vi "manual middle-man to plc barcode print.vi"(8 "error in":errorcluster, 10 "station default states":T1[](array[typedef]) {"LIN INFO"."NAD" format="%.0x"; "LIN INFO"."ADCS LIN"."HW select" items=["NI-XNET", "NI-CAN"]; "LVDT Status"."LVDT's stored config"."Lower Limit" format="%.2f"; "LVDT Status"."LVDT's stored config"."Upper Limit" format="%.2f"; "Store Data"."Sun Shade Open Force Limits"."Variance" format="%.2g"; "Store Data"."Sun Shade Open Force Limits"."Truncation End" format="%.2g"; "Store Data"."Sun Shade Open Force Limits"."Truncation Start" format="%.2g"; "Store Data"."Sun Shade Open Force Limits"."Avg Max" format="%.2g"; "Store Data"."Sun Shade Open Force Limits"."Avg Min" format="%.2g"; "Store Data"."Sun Shade Open Force Limits"."Overall Max" format="%.2g"; "Store Data"."Sun Shade Open Force Limits"."Overall Min" format="%.2g"; "Store Data"."Sun Shade Close Force Limits"."Variance" format="%.2g"; "Store Data"."Sun Shade Close Force Limits"."Truncation End" format="%.2g"; "Store Data"."Sun Shade Close Force Limits"."Truncation Start" format="%.2g"; "Store Data"."Sun Shade Close Force Limits"."Avg Max" format="%.2g"; "Store Data"."Sun Shade Close Force Limits"."Avg Min" format="%.2g"; "Store Data"."Sun Shade Close Force Limits"."Overall Max" format="%.2g"; "Store Data"."Sun Shade Close Force Limits"."Overall Min" format="%.2g"}, 11 "exit program ref":refnum<vi>) -> (0 "error out":errorcluster)   [LabVIEW 2018]
uses:
  05.UserVI's/BarCode/typedefs/barcode printer types.ctl
  05.UserVI's/BarCode/typedefs/barcode format params.ctl
  02.Type Def's/EOL Module Info Control.ctl
  <vilib>/Platform/dataskt.llb/DataSocket Reference Type.ctl
  05.UserVI's/type defs/plc path and tag.ctl
  02.Type Def's/station plc read string tags.ctl
  02.Type Def's/station plc read boolean tags.ctl
  05.UserVI's/type defs/EOL Motor Type.ctl
  05.UserVI's/type defs/RAP Signal Control.ctl
  05.UserVI's/type defs/Communication with Motors.ctl
  02.Type Def's/All Communication Types.ctl
  05.UserVI's/type defs/EOL Part Setup.ctl
  02.Type Def's/All Motions.ctl
  02.Type Def's/EOL Switch Max Min Check Cluster.ctl
  02.Type Def's/EOL Switch Value Configuration Cluster.ctl
  02.Type Def's/All Switch Configuration Cluster.ctl
  05.UserVI's/type defs/17x Sunshade Limts Seq.ctl
  02.Type Def's/Pass Fail Control.ctl
  05.UserVI's/type defs/17x AP Data Type.ctl
  05.UserVI's/type defs/17x Audit Motion Data Seq Control.ctl
  02.Type Def's/EOL Motion Database Table.ctl
  05.UserVI's/sequence/type defs/Sequence Info.ctl
  02.Type Def's/station nvh config.ctl
  02.Type Def's/station rs232 port map.ctl
  02.Type Def's/station ethernet address map.ctl
  02.Type Def's/station paths.ctl
  02.Type Def's/EOL Save Module Test Data Control.ctl
  05.UserVI's/type defs/EOL Global Digital Input Control.ctl
  02.Type Def's/station DI map.ctl
  02.Type Def's/Screen Motion Data.ctl
  02.Type Def's/station motion data indicator.ctl
  02.Type Def's/lvdt name val pair.ctl
  02.Type Def's/station hmi.ctl
  02.Type Def's/individual station status.ctl
  02.Type Def's/control refs.ctl
  05.UserVI's/type defs/EOL LVDT's Check Controller.ctl
  05.UserVI's/Lambda Power/power supply types.ctl
  05.UserVI's/LVDT's/lvdt precision.ctl
  02.Type Def's/main state cluster.ctl
  02.Type Def's/sequence state.ctl
  03.Inalfa LIN/LIN Device.ctl
  <vilib>/CMC.AME/Inalfa ADCS/Ctl'Def/ADCS_LIN info.ctl
  C:/Program Files (x86)/National Instruments/LabVIEW 2018/vi.lib/CMC.AME/_Inalfa TS LIN_internal_deps/Interop.TSMasterAPI.dll
  Program Files (x86)/National Instruments/LabVIEW 2018/vi.lib/CMC.AME/_Inalfa TS LIN_internal_deps/Interop.TSMasterAPI.dll
  02.Type Def's/station LIN config.ctl
  02.Type Def's/misc station config.ctl
  Sub'VIs/Type Def's/Config Info.ctl
panel:
  # "Sunroof Barcode"
  # "Pallet Number"
  # "Part Type"
  # "Application Status"
  # "Current Step"
  # "Cycle Time"
  # "Pass / Fail"
  # "Shade Close"
  # "Actual Data"
  # "Limits"
  # "Avg Current"
  # "Run Time"
  # "Speed"
  # "Noise Test"
  # "Position"
  # "Shade Open"
  # "Actual Data"
  # "Limits"
  # "Avg Current"
  # "Run Time"
  # "Speed"
  # "Noise Test"
  # "Position"
  # "Vent Close"
  # "Actual Data"
  # "Limits"
  # "Avg Current"
  # "Run Time"
  # "Speed"
  # "Noise Test"
  # "Position"
  # "Vent Open"
  # "Actual Data"
  # "Limits"
  # "Avg Current"
  # "Run Time"
  # "Speed"
  # "Noise Test"
  # "Position"
  # "Slide Close"
  # "Actual Data"
  # "Limits"
  # "Avg Current"
  # "Run Time"
  # "Speed"
  # "Noise Test"
  # "Position"
  # "Slide Open"
  # "Actual Data"
  # "Limits"
  # "Avg Current"
  # "Run Time"
  # "Speed"
  # "Noise Test"
  # "Position"
  # "Min"
  # "N"
  # "Min"
  # "Start"
  # "N"
  # "Max"
  # "N"
  # "Max"
  # "N"
  # "End"
  # "Min"
  # "N"
  # "Min"
  # "Start"
  # "N"
  # "Max"
  # "N"
  # "Max"
  # "N"
  # "End"
  # "Min"
  # "Max"
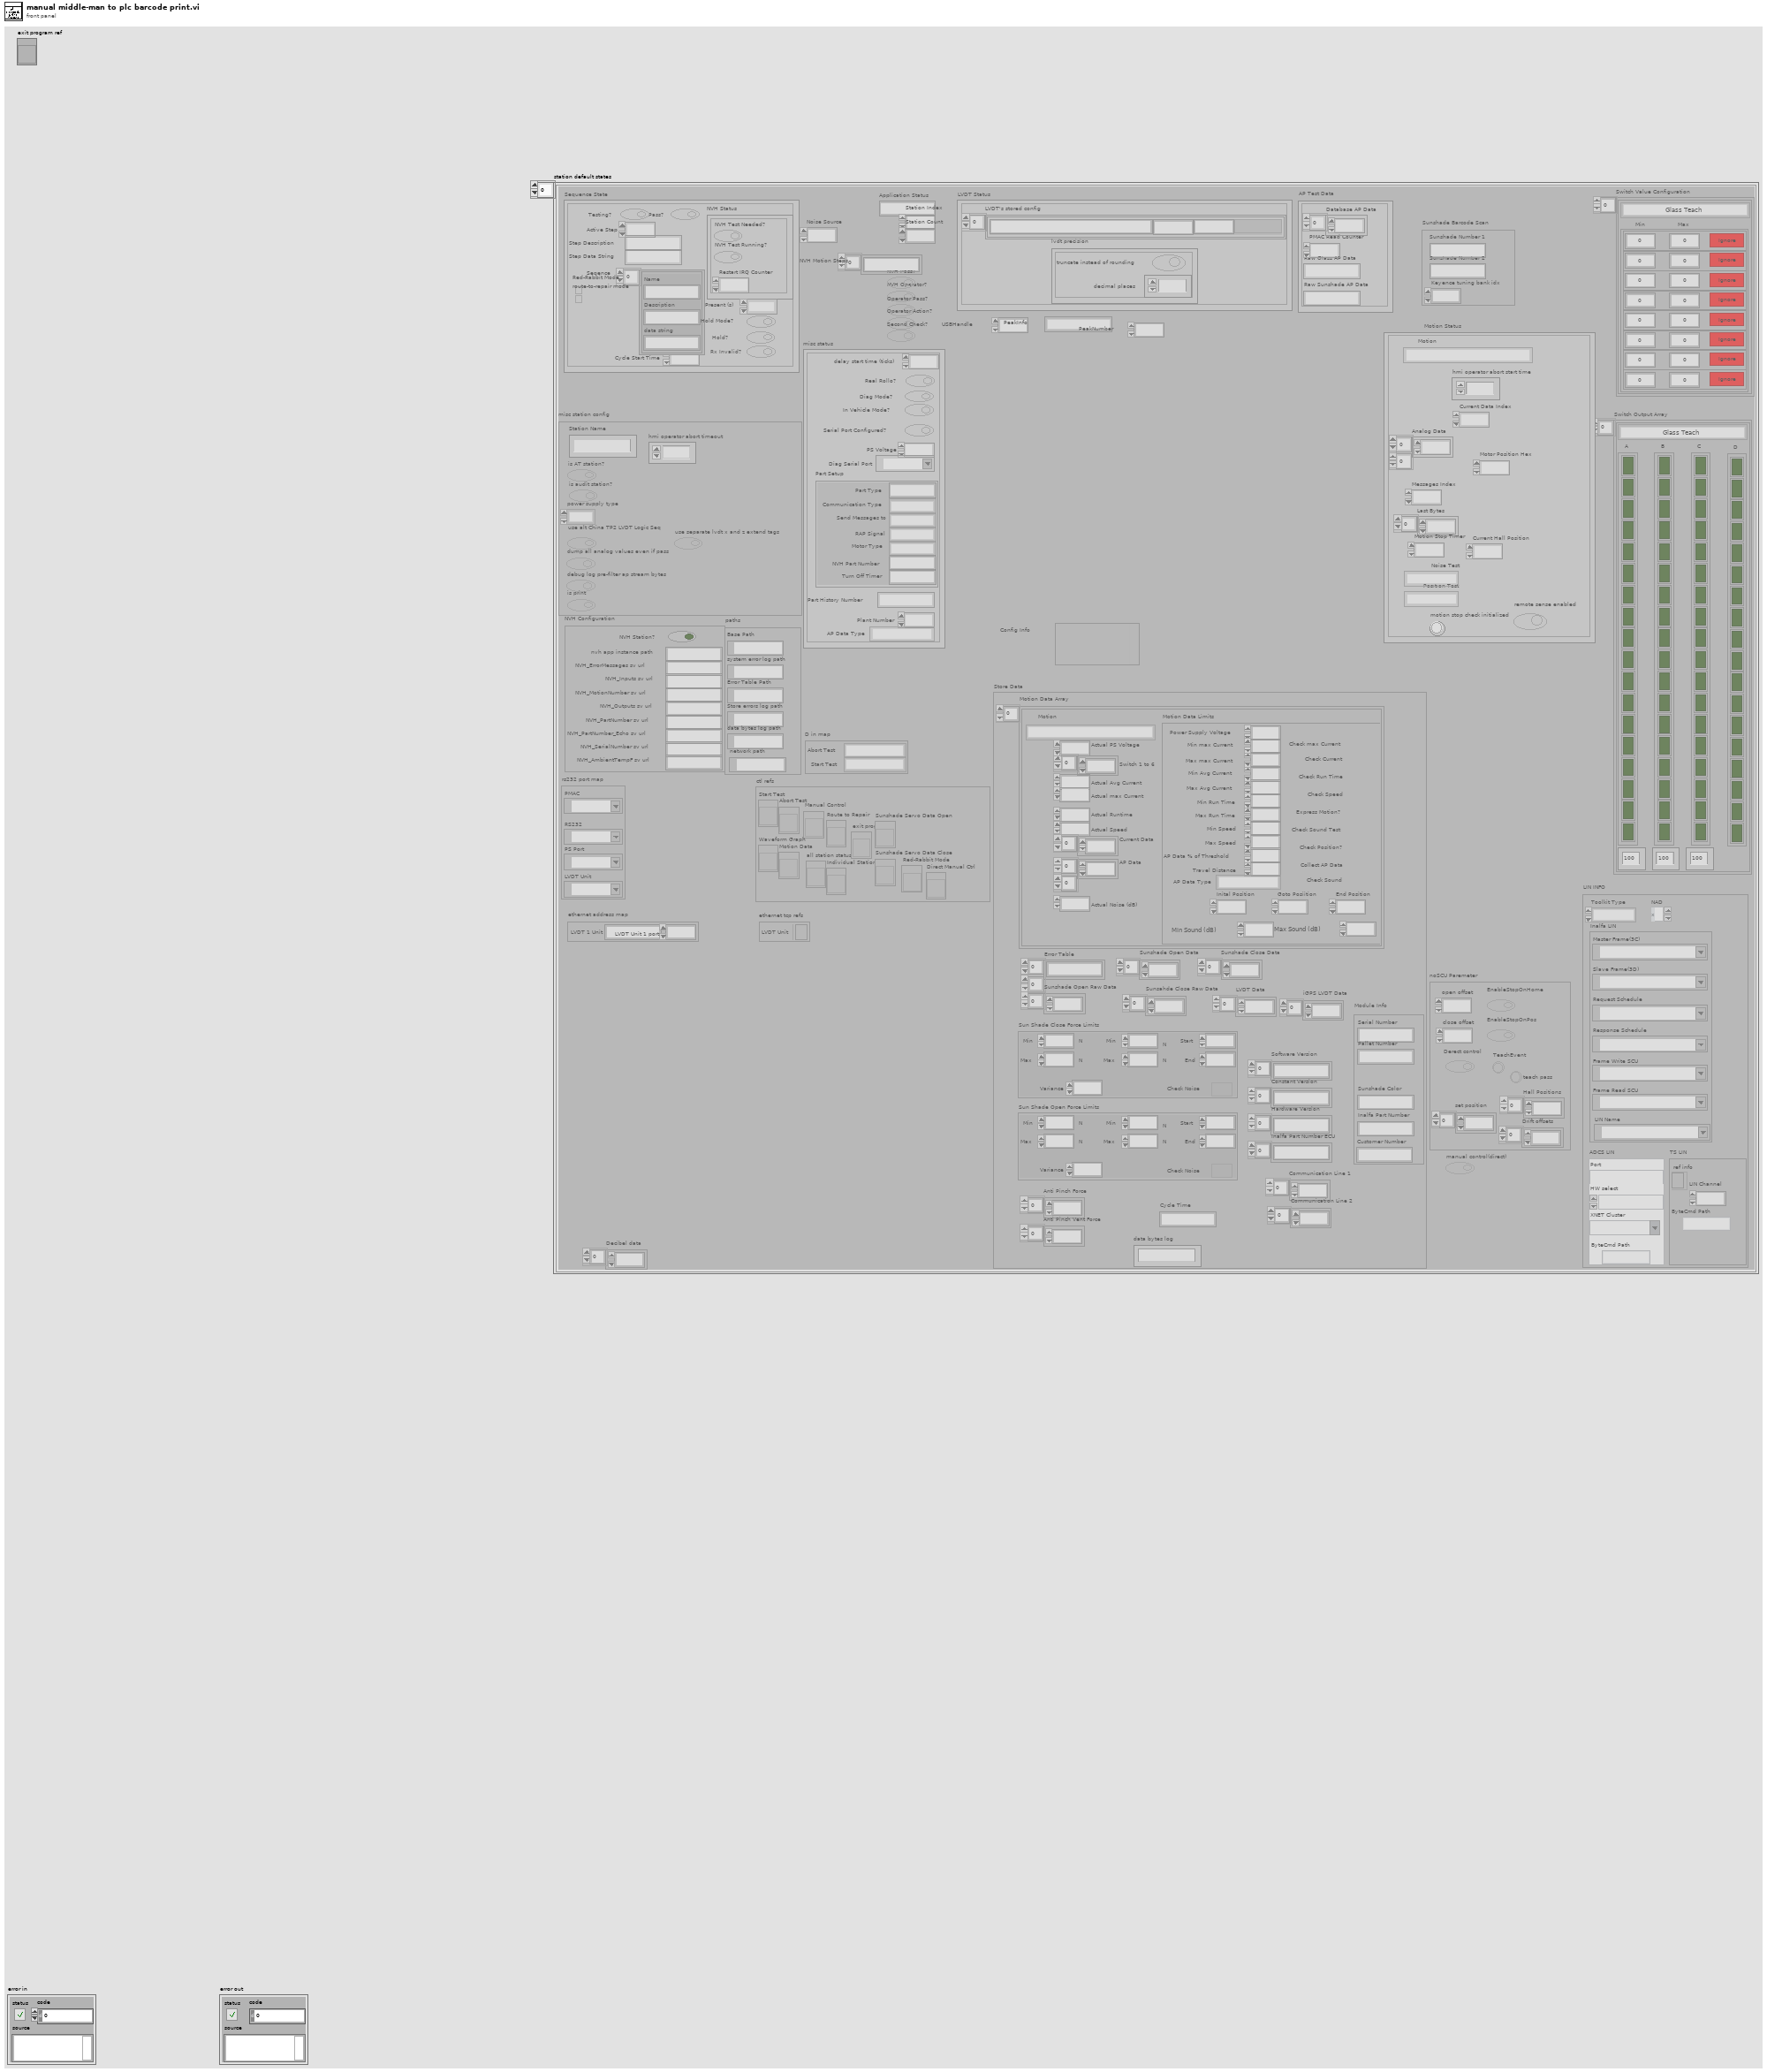
[diagram p1: front panel]
types:
  T1 = typedef "main state cluster.ctl" = cluster{"Application Status":string, "Switch Output Array":T2[], "Switch Value Configuration":T4[], "NVH Configuration":T6, "rs232 port map":T7, "ethernet address map":T8, "paths":T9, "Station Index":i32, "Station Count":i32, "Store Data":T10, "D in map":T16, "ctl refs":T18, "misc station config":T19, "ethernet tcp refs":cluster{"LVDT Unit":refnum<k5>}, "Sunshade Barcode Scan":cluster{"Sunshade Number 2":string, "Sunshade Number 1":string, "Keyence tuning bank idx":i32}, "AP Test Data":cluster{"Raw Sunshade AP Data":string, "Raw Glass AP Data":string, "PMAC Read Counter":dbl, "Database AP Data":dbl[]}, "Motion Status":cluster{"hmi operator abort start time":u32, "Current Data Index":i32, "Analog Data":sgl[][], "Motor Position Hex":u16, "Messages Index":u16, "Last Bytes":u8[], "Current Hall Position":i16, "Motion Stop Timer":u32, "Position Test":T21, "Noise Test":T21, "motion stop check initialized":bool, "remote sense enabled":bool, "Motion":T3}, "LVDT Status":cluster{"LVDT's stored config":T22[], "lvdt precision":T23}, "Sequence State":T24, "misc status":cluster{"delay start time (ticks)":u32, "In Vehicle Mode?":bool, "Diag Mode?":bool, "Serial Port Configured?":bool, "PS Voltage":dbl, "Diag Serial Port":refnum<visa-resource-name>, "Part Setup":T26, "Part History Number":string, "Plant Number":u8, "AP Data Type":T13, "Real Rollo?":bool}, "NVH Operator?":bool, "NVH Pass?":bool, "Operator Pass?":bool, "Operator Action?":bool, "Noise Source":u32, "USBHandle":i32, "PeakInfo":string, "PeakNumber":i32, "NVH Motion Steps":string[], "Second Check?":bool, "Decibel data":dbl[], "noSCU Paremeter":cluster{"EnableStopOnHome":bool, "EnableStopOnPos":bool, "TeachEvent":bool, "open offset":i32, "close offset":i32, "Derect control":bool, "set position":i32[], "teach pass ":bool, "Drift offsets":i32[], "Hall Positions":i32[]}, "manual control(direct)":bool, "LIN INFO":T31, "Config Info":T34}
  T2 = typedef "All Switch Configuration Cluster.ctl" = cluster{"All Motions":T3, "A":bool[], "B":bool[], "C":bool[], "D":bool[], "A activation time (ms)":u32, "B activation time (ms)":u32, "C activation time (ms)":u32}
  T3 = typedef "All Motions.ctl" = enum16{"Glass Teach", "Glass Slide Open", "Glass Slide Close", "Glass Vent Open", "Glass Vent Close", "Sunshade Teach", "Sunshade Open", "Sunshade Close", "Idle", "Sunshade Open 2", "Sunshade Close 2", "Glass Slide Open Sunshade Open", "Glass Slide Open Sunshade Close", "Glass Slide Close Sunshade Open", "Glass Slide Close Sunshade Close", "Glass Vent Open Sunshade Open", "Glass Vent Open Sunshade Close", "Glass Vent Close Sunshade Open", "Glass Vent Close Sunshade Close", "Express Glass Slide Open", "Express Glass Slide Close", "Express Glass Vent Open", "Express Glass Vent Close", "Express Sunshade Open", "Express Sunshade Close", "Express Sunshade Open 2", "Express Sunshade Close 2", "Express Glass Slide Open Sunshade Open", "Express Glass Slide Open Sunshade Close", "Express Glass Slide Close Sunshade Open", "Express Glass Slide Close Sunshade Close", "Express Glass Vent Open Sunshade Open", "Express Glass Vent Open Sunshade Close", "Express Glass Vent Close Sunshade Open", "Express Glass Vent Close Sunshade Close", "Goto Position Glass", "Goto Position Sunshade", "Sunshade Teach 2"}
  T4 = typedef "EOL Switch Value Configuration Cluster.ctl" = cluster{"All Motions":T3, "Array":T5[]}
  T5 = typedef "EOL Switch Max Min Check Cluster.ctl" = cluster{"Min":dbl, "Max":dbl, "Check?":bool}
  T6 = typedef "station nvh config.ctl" = cluster{"NVH Station?":bool, "nvh app instance path":string, "NVH_ErrorMessages sv url":string, "NVH_Inputs sv url":string, "NVH_MotionNumber sv url":string, "NVH_Outputs sv url":string, "NVH_PartNumber sv url":string, "NVH_PartNumber_Echo sv url":string, "NVH_SerialNumber sv url":string, "NVH_AmbientTempF sv url":string}
  T7 = typedef "station rs232 port map.ctl" = cluster{"PMAC":refnum<visa-resource-name>, "PS Port":refnum<visa-resource-name>, "LVDT Unit":refnum<visa-resource-name>, "RS232":refnum<visa-resource-name>}
  T8 = typedef "station ethernet address map.ctl" = cluster{"LVDT 1 Unit":string, "LVDT Unit 1 port":u16}
  T9 = typedef "station paths.ctl" = cluster{"Base Path":path, "system error log path":path, "Error Table Path":path, "Store errors log path":path, "data bytes log path":path, "network path":path}
  T10 = typedef "EOL Save Module Test Data Control.ctl" = cluster{"Motion Data Array":T11[], "Error Table":string[][], "Sun Shade Close Force Limits":T14, "Sun Shade Open Force Limits":T14, "Sunshade Open Data":sgl[], "Sunshade Close Data":sgl[], "Module Info":T15, "Sunsahde Close Raw Data":sgl[], "Sunshade Open Raw Data":sgl[], "Software Version":string[], "Constant Version":string[], "Hardware Version":string[], "Inalfa Part Number ECU":string[], "LVDT Data":sgl[], "Communication Line 1":sgl[], "Communication Line 2":sgl[], "Anti Pinch Force":sgl[], "Cycle Time":string, "Anti Pinch Vent Force":sgl[], "iGPS LVDT Data":sgl[], "data bytes log":string}
  T11 = typedef "EOL Motion Database Table.ctl" = cluster{"Motion":T3, "Actual Avg Current":dbl, "Actual Runtime":dbl, "Actual Speed":dbl, "Current Data":sgl[], "Motion Data Limits":T12, "Switch 1 to 6":dbl[], "Actual PS Voltage":dbl, "AP Data":i16[][], "Actual max Current":dbl, "Actual Noise (dB)":dbl}
  T12 = typedef "17x Audit Motion Data Seq Control.ctl" = cluster{"Power Supply Voltage":dbl, "Min Avg Current":dbl, "Max Avg Current":dbl, "Min Run Time":dbl, "Max Run Time":dbl, "Min Speed":dbl, "Max Speed":dbl, "AP Data % of Threshold":dbl, "Travel Distance":dbl, "AP Data Type":T13, "Check Current":bool, "Check Run Time":bool, "Check Speed":bool, "Express Motion?":bool, "Check Sound Test":bool, "Check Position?":bool, "Collect AP Data":bool, "Inital Position":u16, "End Position":u16, "Goto Posiition":u16, "Max max Current":dbl, "Min max Current":dbl, "Check max Current":bool, "Check Sound":bool, "Min Sound (dB)":dbl, "Max Sound (dB)":dbl}
  T13 = typedef "17x AP Data Type.ctl" = enum16{"91/61", "92/62", "93/63", "67", "68", "6F", "71", "91 Msg", "92 Msg", "93 Msg", "94 Msg", "HiRain 91", "HiRain 92 Speed", "HiRain 92 HS", "HiRain 92", "HiRain 93", "SnT"}
  T14 = typedef "17x Sunshade Limts Seq.ctl" = cluster{"Overall Min":dbl, "Overall Max":dbl, "Avg Min":dbl, "Avg Max":dbl, "Truncation Start":dbl, "Truncation End":dbl, "Variance":dbl, "Check Noise":bool}
  T15 = typedef "EOL Module Info Control.ctl" = cluster{"Serial Number":string, "Pallet Number":string, "Sunshade Color":string, "Inalfa Part Number":string, "Customer Number":string}
  T16 = typedef "station DI map.ctl" = cluster{"Abort Test":T17, "Start Test":T17}
  T17 = typedef "EOL Global Digital Input Control.ctl" = enum16{"Dev2/port0/line0", "Dev2/port0/line1", "Dev2/port0/line2", "Dev2/port0/line3", "Dev2/port0/line4", "Dev2/port0/line5", "Dev2/port0/line6", "Dev2/port0/line7", "Dev2/port1/line0", "Dev2/port1/line1", "Dev2/port1/line2", "Dev2/port1/line3", "Dev2/port1/line4", "Dev2/port1/line5", "Dev2/port1/line6", "Dev2/port1/line7", "Dev2/port2/line0", "Dev2/port2/line1", "Dev2/port2/line2", "Dev2/port2/line3", "Dev2/port2/line4", "Dev2/port2/line5", "Dev2/port2/line6", "Dev2/port2/line7", "Prerun Start Test", "Prerun Abort Test", "Audit Start Test", "Audit Abort Test", "Dev2/port3/line4", "Dev2/port3/line5", "Breakin Start Test", "Breakin Abort Test", "Not Implemented"}
  T18 = typedef "control refs.ctl" = cluster{"Start Test":refnum<vi>, "Abort Test":refnum<vi>, "Manual Control":refnum<vi>, "Route to Repair":refnum<vi>, "Waveform Graph":refnum<vi>, "Motion Data":refnum<vi>, "all station status":refnum<vi>, "Individual Station Status":refnum<vi>, "exit program":refnum<vi>, "Sunshade Servo Data Open":refnum<vi>, "Sunshade Servo Data Close":refnum<vi>, "Red-Rabbit Mode":refnum<vi>, "Direct Manual Ctrl":refnum<vi>}
  T19 = typedef "misc station config.ctl" = cluster{"Station Name":string, "is AT station?":bool, "is audit station?":bool, "power supply type":T20, "use alt China TP2 LVDT Logic Seq":bool, "hmi operator abort timeout":u32, "dump all analog values even if pass":bool, "debug log pre-filter ap stream bytes":bool, "use separate lvdt x and z extend tags":bool, "is print":bool}
  T20 = typedef "power supply types.ctl" = enum16{"GENser", "ZUPser", "GENeth", "Manual", "ITECH"}
  T21 = typedef "Pass Fail Control.ctl" = enum16{"Not Tested", "Pass", "Fail"}
  T22 = typedef "EOL LVDT's Check Controller.ctl" = cluster{"Upper Limit":dbl, "Lower Limit":dbl, "LVDT Name":string, "Check":bool}
  T23 = typedef "lvdt precision.ctl" = cluster{"truncate instead of rounding":bool, "decimal places":u8}
  T24 = typedef "sequence state.ctl" = cluster{"Step Description":string, "Cycle Start Time":u32, "Step Data String":string, "Pass?":bool, "Seqence":T25[], "Active Step":u8, "Testing?":bool, "Red-Rabbit Mode":bool, "route-to-repair mode":bool, "NVH Status":cluster{"Restart IRQ Counter":u8, "NVH Test Needed?":bool, "NVH Test Running?":bool}, "Present (s)":dbl, "Hold Mode?":bool, "Hold?":bool, "Rx Invalid?":bool}
  T25 = typedef "Sequence Info.ctl" = cluster{"Name":string, "Description":string, "data string":string}
  T26 = typedef "EOL Part Setup.ctl" = cluster{"Communication Type":T27, "Send Messages to":T28, "RAP Signal":T29, "Motor Type":T30, "NVH Part Number":u16, "Turn Off Timer":u16, "Part Type":string}
  T27 = typedef "All Communication Types.ctl" = enum16{"None", "CAN", "RS 232", "RS 232 LIN", "GM LIN", "SnT LIN", "K Line", "Robel CAN", "P42M-Continental", "Inalfa SCU LIN", "Spare 3"}
  T28 = typedef "Communication with Motors.ctl" = enum16{"Glass", "Rollo", "Both"}
  T29 = typedef "RAP Signal Control.ctl" = enum16{"High", "Low", "None"}
  T30 = typedef "EOL Motor Type.ctl" = enum16{"Smart Motor", "Sensor Motor"}
  T31 = typedef "station LIN config.ctl" = cluster{"Toolkit Type":enum16{"Inalfa LIN", "ADCS LIN", "TS LIN"}, "NAD":u8, "Inalfa LIN":T32, "ADCS LIN":T33, "TS LIN":cluster{"ref info":refnum<k24>, "LIN Channel":i32, "ByteCmd Path":path}}
  T32 = typedef "LIN Device.ctl" = cluster{"Master Frame(3C)":refnum<k21>, "Slave Frame(3D)":refnum<k21>, "Request Schedule":refnum<k21>, "Response Schedule":refnum<k21>, "Frame Write SCU":refnum<k21>, "Frame Read SCU":refnum<k21>, "LIN Name":refnum<k21>}
  T33 = typedef "ADCS_LIN info.ctl" = cluster{"Port":string, "HW select":u16, "XNET Cluster":string, "ByteCmd Path":path}
  T34 = typedef "Config Info.ctl" = variant
  T35 = typedef "station plc read boolean tags.ctl" = cluster{"AT glass position":T36, "AT shade position":T36, "AT in glass wand lower pos":T36, "AT in sunshad wand lower pos":T36, "AT in wand home pos":T36, "LVDT's Extended":T36, "motor foam present LH":T36, "motor foam present RH":T36, "audit gap hider present LH":T36, "audit gap hider present RH":T36, "FB light block present":T36, "bolt check 1":T36, "bolt check 2":T36, "bolt check 3":T36, "bolt check 4":T36, "bolt check 5":T36, "bolt check 6":T36, "bolt check 7":T36, "bolt check 8":T36, "bolt check 9":T36, "bolt check 10":T36, "bolt check 11":T36, "bolt check 12":T36, "bolt check 13":T36, "bolt check 14":T36, "bolt check 15":T36, "bolt check 16":T36, "bolt check 17":T36, "bolt check 18":T36, "bolt check 19":T36, "bolt check 20":T36, "bolt check 21":T36, "start":T36, "abort":T36, "LVDT's Retracted":T36, "manual barcode print":T36, "ss servo at open":T36, "ss servo at close":T36, "ss servo opening":T36, "ss servo closing":T36, "control slide at home":T36, "control slide left good":T36, "control slide left over stroke":T36, "control slide right good":T36, "control slide right over stroke":T36, "wind deflector high speed pos":T36, "wind deflector low speed pos":T36, "AT VentPMACatHome":T36, "AT VentPMACisExtend":T36, "SS Barcode Scanner Bypassed":T36, "Check Frame Barcode":T36, "iGPS Pass 0":T36, "iGPS Pass 1":T36, "iGPS Pass 2":T36, "iGPS Pass 3":T36, "iGPS Pass 4":T36, "iGPS Pass 5":T36, "iGPS Pass 6":T36, "iGPS Pass 7":T36, "iGPS Pass 8":T36, "iGPS Pass 9":T36, "Z LVDTs Extended":T36, "NVH Operator Pass":T36, "NVH Operator Fail":T36, "NVH Operator Express Glass Open":T36, "NVH Operator Express Glass Close":T36, "NVH Operator Express Rollo Open01":T36, "NVH Operator Express Rollo Close01":T36, "NVH Operator Express Rollo Open02":T36, "NVH Operator Express Rollo Close02":T36, "NVH Operator Vent Open Noise":T36, "NVH Operator Vent Close Noise":T36, "NVH Operator Sunshade Open Noise":T36, "NVH Operator Sunshade Close Noise":T36, "NVH Operator Glass Open Noise":T36, "NVH Operator Glass Close Noise":T36, "NVH Operator Finish":T36, "NVH Operator Check":T36, "AT shade 02 position":T36, "AT in sunshad 02 wand up pos":T36, "AT in wand 02 home pos":T36, "windproof position":T36, "NVH Operator Express Glass vent Open":T36, "NVH Operator Express Glass Vent Close":T36, "NVH Operator Re-do":T36, "AT at vent ATS test pos":T36, "AT at vent ATS Home pos":T36, "Start Adjust LVDT":T36, "Finish Adjust LVDT":T36}
  T36 = typedef "plc path and tag.ctl" = cluster{"Tag Name":string, "Network Path":string, "use opc":bool, "DataSocket Reference":T37}
  T37 = typedef "DataSocket Reference Type.ctl" = cluster{"CWDSLib._DCWDataSocket":refnum<k7>, "CWDSLib._DCWData":refnum<k7>, "OnDataUpdated":u32, "OnStatusUpdated":u32}
  T38 = typedef "station plc read string tags.ctl" = cluster{"Serial Number":T36, "Pallet Number":T36, "Inalfa Part Number":T36, "Shade Color":T36, "Model Type":T36, "Customer Number":T36, "Part History Number":T36, "Shade 1 Barcode":T36, "Shade 2 Barcode":T36, "Manual Serial Number":T36, "Manual Inalfa Part Number":T36, "Manual Shade Color":T36, "Manual Model Type":T36, "Manual Customer Number":T36, "Manual Part History Number":T36, "iGPS SN 0":T36, "iGPS SN 1":T36, "iGPS SN 2":T36, "iGPS SN 3":T36, "iGPS SN 4":T36, "iGPS SN 5":T36, "iGPS SN 6":T36, "iGPS SN 7":T36, "iGPS SN 8":T36, "iGPS SN 9":T36}
  T39 = cluster{"St 60 MBC Print":bool, "St 100 MBC Print":bool, "Module Info":T15, "PHN":string, "st60 PLC read boolean Tags":T35, "st60 PLC string read Tags":T38, "st100 PLC string read Tags":T38, "st100 PLC read boolean Tags":T35, "paths.Base Path":path, "Exit Program":refnum<vi>, "Part Type":string}
  T40 = typedef "WKLXF25 St 60 PLC Data Control.ctl" = cluster{"Serial Number":string, "Inalfa Part Number":string, "Sunshade Color":string, "Shade 1 Barcode":string, "Shade 2 Barcode":string, "Model Type":string, "Part History Number":string, "Customer Number":string}
  T41 = typedef "barcode format params.ctl" = cluster{"Format String":string, "Print String":string, "Quantity":u8, "printer type":T42, "RS232 Port":string, "IP Address":string, "Ethernet Port":u32}
  T42 = typedef "barcode printer types.ctl" = enum16{"Intermec RS232", "Intermec Ethernet"}
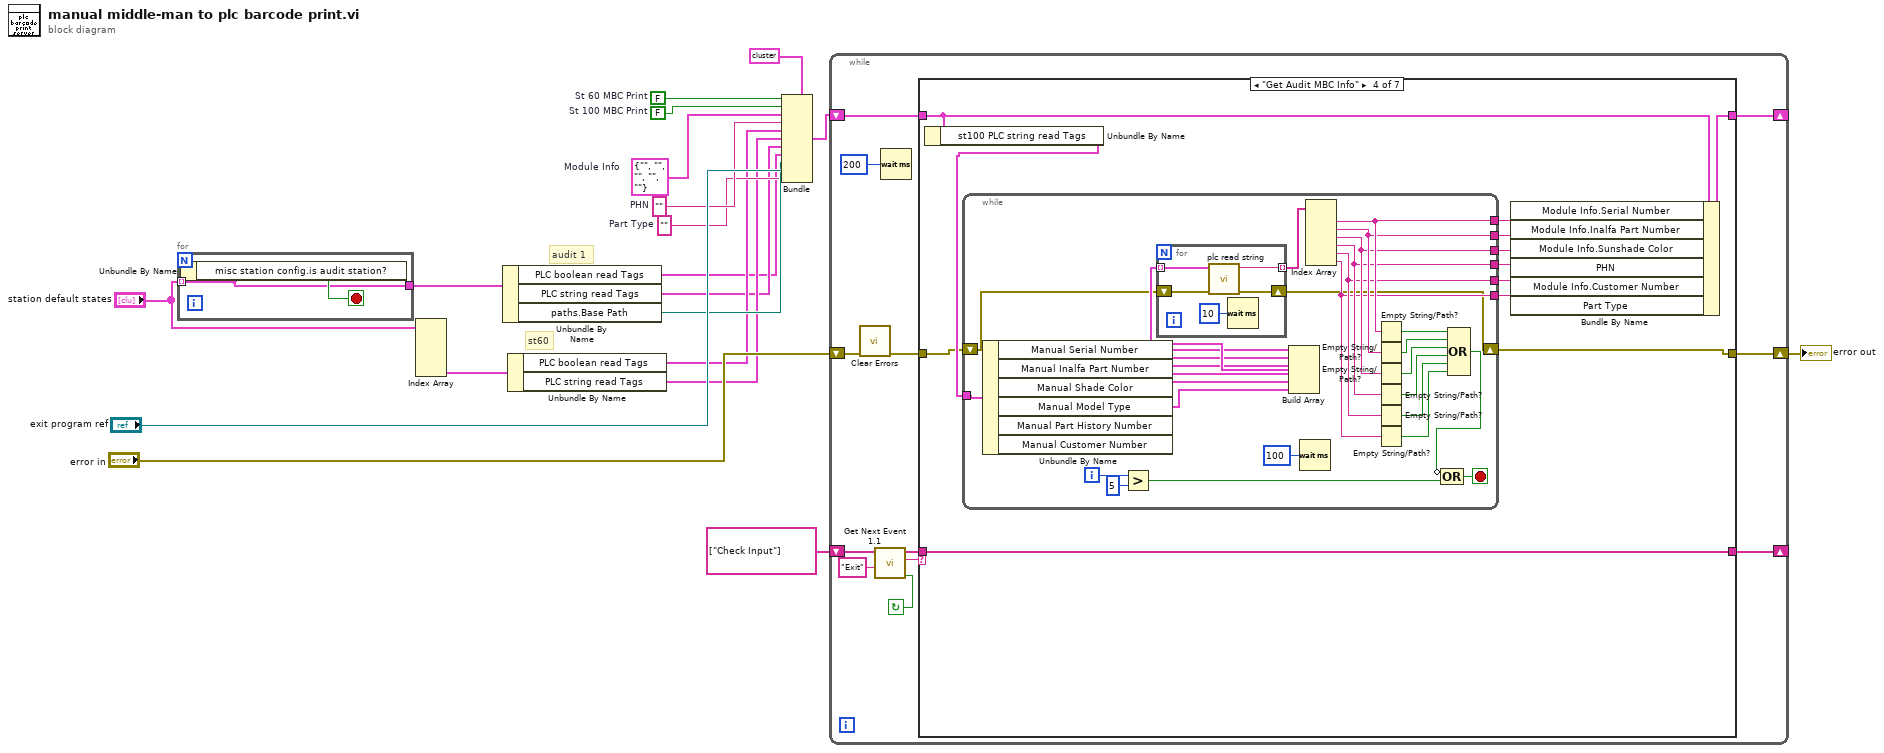
[diagram p0: block diagram]
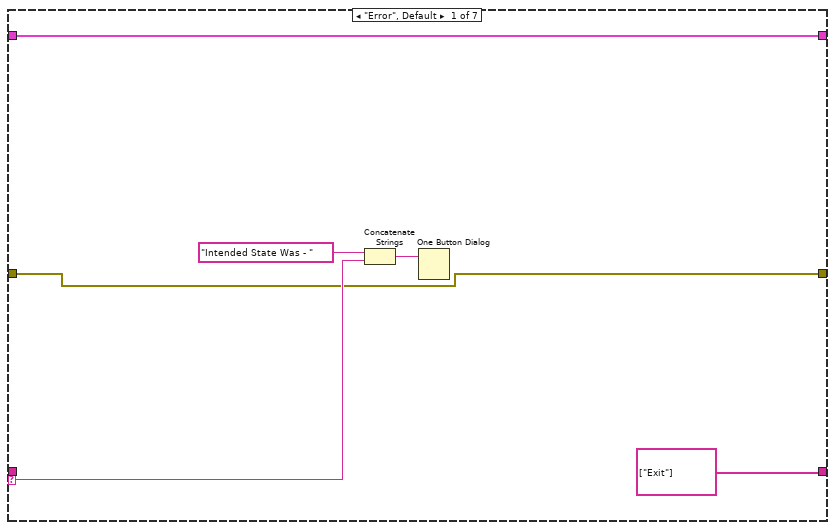
[diagram p2: hidden frame]
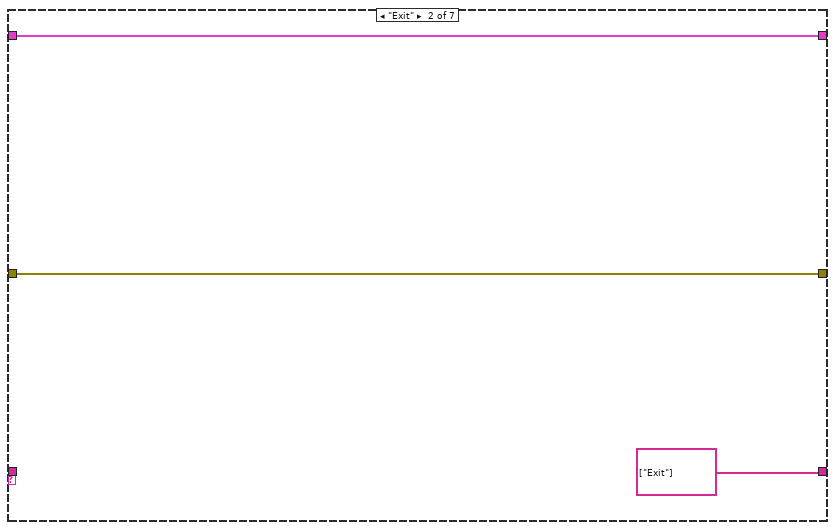
[diagram p3: hidden frame]
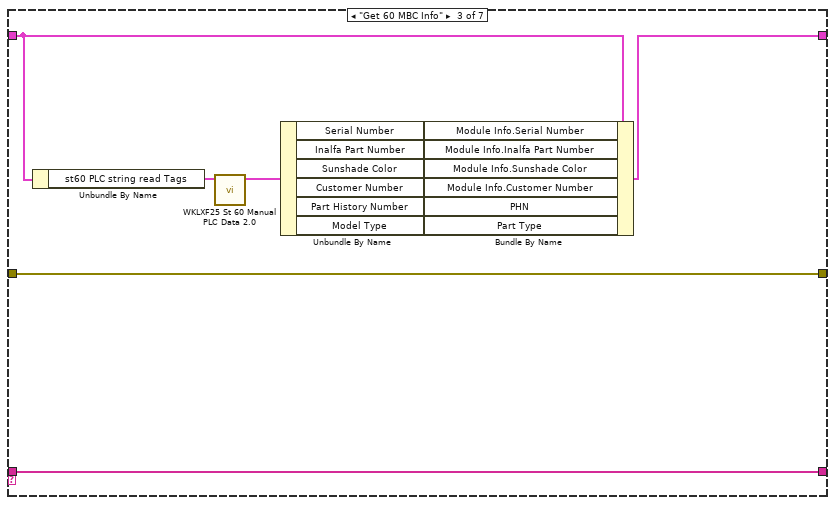
[diagram p4: hidden frame]
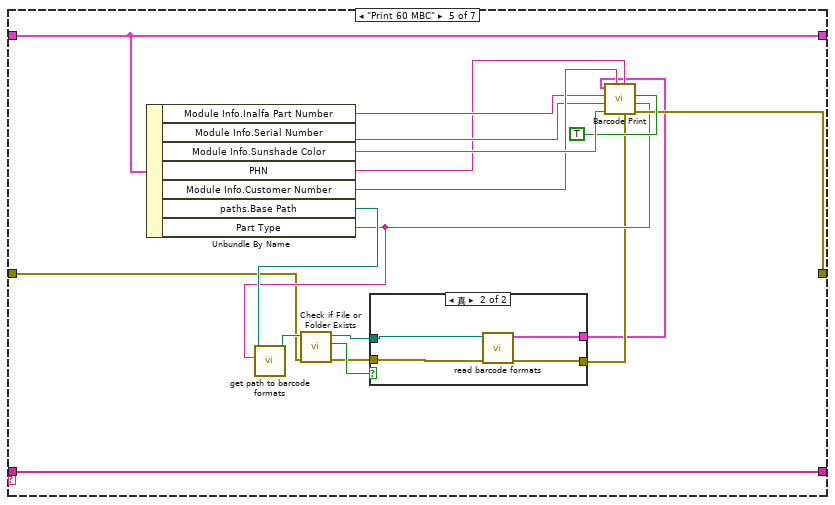
[diagram p5: hidden frame]
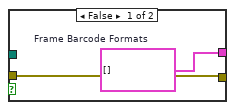
[diagram p6: hidden frame]
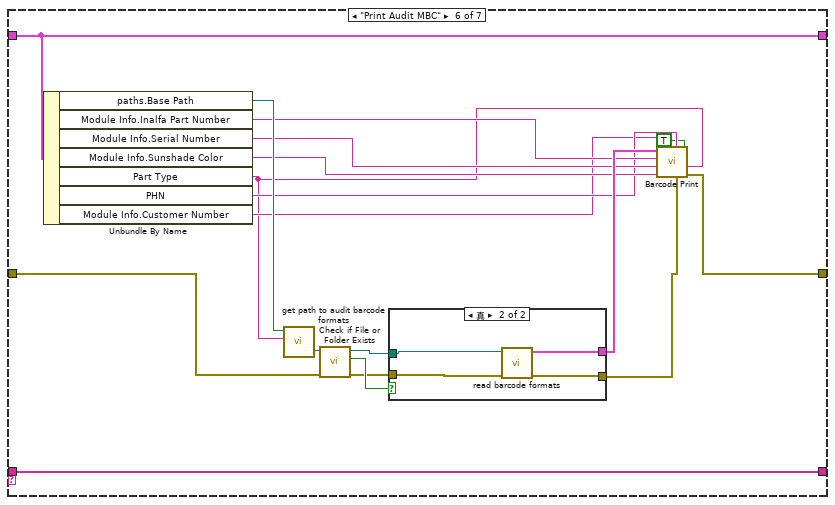
[diagram p7: hidden frame]
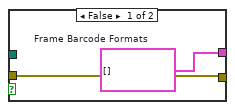
[diagram p8: hidden frame]
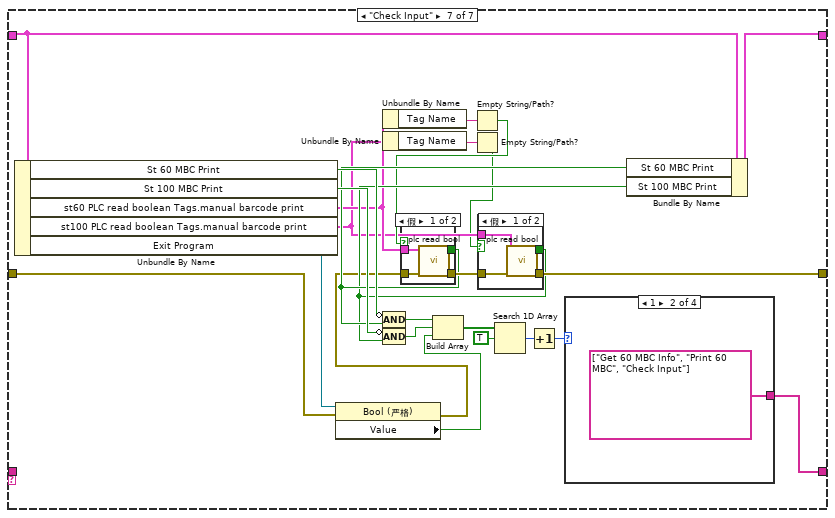
[diagram p9: hidden frame]
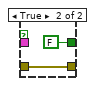
[diagram p10: hidden frame]
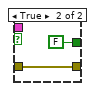
[diagram p11: hidden frame]
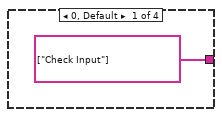
[diagram p12: hidden frame]
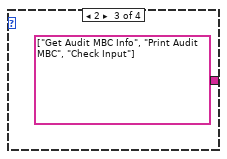
[diagram p13: hidden frame]
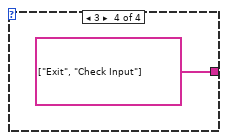
[diagram p14: hidden frame]
diagram:
  w5 = ""  # Part Type
  w13 = ""  # PHN
  w12 = T15 {"Serial Number"="", "Pallet Number"="", "Sunshade Color"="", "Inalfa Part Number"="", "Customer Number"=""}  # Module Info
  w10 = FALSE  # St 100 MBC Print
  w9 = FALSE  # St 60 MBC Print
  # "st60"
  # "audit 1"
  n1 = for {
    tunnel: "station default states" -> [w20] mode=indexing
    tunnel: [w20] -> w16
    stop <- w21 stop-if-true
    n2 = Unbundle By Name(w20) -> ("misc station config.is audit station?"=w21:bool)
  }
  n3 = Index Array(array="station default states") -> (element #5=w14:T1)  [unwired: 5 in, 4 out]
  n4 = Unbundle By Name(w16) -> ("PLC boolean read Tags"=w1:T35, "PLC string read Tags"=w2:T38, "paths.Base Path"=w18:path)
  n5 = Unbundle By Name(w14) -> ("PLC boolean read Tags"=w4:T35, "PLC string read Tags"=w3:T38)
  n6 = Bundle(cluster=T39 data[5746B], "St 60 MBC Print"=w9, "St 100 MBC Print"=w10, "Module Info"=w12, "PHN"=w13, "st60 PLC read boolean Tags"=w4, "st60 PLC string read Tags"=w3, "st100 PLC string read Tags"=w2, "st100 PLC read boolean Tags"=w1, "paths.Base Path"=w18, "Exit Program"="exit program ref", "Part Type"=w5) -> (w11:T39)
  n7 = while {
    shift-right: [w29] -> _
    shift-left: string[] ["Check Input"] ("event queue out") -> [w28]
    shift-right: [w26] -> _
    shift-left: w11 -> [w27]
    shift-right: [w24] -> w6
    shift-left: "error in" -> [w23]
    stop <- w33 continue-if-true
    n8 = call <vilib>:"Clear Errors.vi"("error in (no error)"=w23) -> ("error out"=w25:errorcluster)  [unwired: 5 in, 1 out]
    n9 = call "Get Next Event 1.1.vi"("Exit Event"="Exit", "event queue in"=w28) -> ("Condition (Exit:F)"=w33:bool, "next event"=w31:string, "event queue out"=w30:string[])  [unwired: 6 in, 1 out]
    n10 = Wait (ms)(milliseconds to wait=u32 200) -> ()  [unwired: 1 out]
    n11 = case shown="\"Get Audit MBC Info\"" w31 {
      selector: w31 -> [w38 _ _ _ _ _ _]
      tunnel: w30 -> [_ _ w54 w66 w118 w142 _]
      tunnel: [string[] ["Exit"] ("event queue out") string[] ["Exit"] ("event queue out") w54 w66 w118 w142 w169] -> w29
      tunnel: w27 -> [w35 w41 w45 w58 w110 w141 w166]
      tunnel: [w35 w41 w53 w62 w110 w141 w165] -> w26
      tunnel: w25 -> [w34 w40 w43 w56 w103 w135 w157]
      tunnel: [w34 w40 w43 w55 w111 w127 w160] -> w24
      frame "Error", Default {
        n12 = Concatenate Strings("Intended State Was - " ("string"), w38) -> (w37:string)
        n13 = One Button Dialog(message=w37) -> ()  [unwired: 1 in, 1 out]
      }
      frame "Exit" {
      }
      frame "Get 60 MBC Info" {
        n14 = Unbundle By Name(w45) -> ("st60 PLC string read Tags"=w44:T38)
        n15 = call "WKLXF25 St 60 Manual PLC Data 2.0.vi"("station plc read string tags"=w44) -> ("PLC Data"=w52:T40)  [unwired: 6 in, 2 out]
        n16 = Unbundle By Name(w52) -> ("Serial Number"=w51:string, "Inalfa Part Number"=w50:string, "Sunshade Color"=w49:string, "Customer Number"=w48:string, "Part History Number"=w47:string, "Model Type"=w46:string)
        n17 = Bundle By Name(cluster=w45, "Module Info.Serial Number"=w51, "Module Info.Inalfa Part Number"=w50, "Module Info.Sunshade Color"=w49, "Module Info.Customer Number"=w48, "PHN"=w47, "Part Type"=w46) -> (w53:T39)
      }
      frame "Get Audit MBC Info" {
        n18 = Unbundle By Name(w58) -> ("st100 PLC string read Tags"=w57:T38)
        n19 = while {
          tunnel: [w85] -> w65
          tunnel: [w84] -> w64
          tunnel: [w83] -> w63
          tunnel: [w82] -> w61
          tunnel: [w79] -> w60
          tunnel: [w78] -> w59
          tunnel: w57 -> [w69]
          shift-right: [w67] -> w55
          shift-left: w56 -> [w68]
          i -> [w94]
          stop <- w91 stop-if-true
          n20 = Unbundle By Name(w69) -> ("Manual Serial Number"=w74:T36, "Manual Inalfa Part Number"=w75:T36, "Manual Shade Color"=w76:T36, "Manual Model Type"=w70:T36, "Manual Part History Number"=w72:T36, "Manual Customer Number"=w71:T36)
          n21 = Greater?(x=w94, y=5) -> (0:w92:bool)
          n22 = Build Array(w74, w75, w76, w72, w71, w70) -> (w77:T36[])
          n23 = for {
            tunnel: w77 -> [w100] mode=indexing
            shift-right: [w97] -> w67
            shift-left: w68 -> [w99]
            tunnel: [w98] -> w73 mode=indexing
            n24 = call "plc read string.vi"("error in"=w99, "addr,tag"=w100) -> ("error out"=w97:errorcluster, "Data"=w98:string)  [unwired: 8 in]
            n25 = Wait (ms)(milliseconds to wait=u32 10) -> ()  [unwired: 1 out]
          }
          n26 = Wait (ms)(milliseconds to wait=u32 100) -> ()  [unwired: 1 out]
          n27 = Index Array(array=w73) -> (element #1=w85:string, element #2=w84:string, element #3=w83:string, element #4=w82:string, element #5=w79:string, element #6=w78:string)  [unwired: 6 in]
          n28 = Empty String/Path?(string/path=w85) -> (empty?=w89:bool)
          n29 = Empty String/Path?(string/path=w84) -> (empty?=w90:bool)
          n30 = Empty String/Path?(string/path=w83) -> (empty?=w87:bool)
          n31 = Empty String/Path?(string/path=w82) -> (empty?=w86:bool)
          n32 = Empty String/Path?(string/path=w79) -> (empty?=w81:bool)
          n33 = Empty String/Path?(string/path=w78) -> (empty?=w80:bool)
          n34 = Compound Arithmetic op=OR(w89, w90, w87, w86, w81, w80) -> (w88:bool)
          n35 = Compound Arithmetic op=OR(invert w88, w92) -> (w91:bool)
        }
        n36 = Bundle By Name(cluster=w58, "Module Info.Serial Number"=w65, "Module Info.Inalfa Part Number"=w64, "Module Info.Sunshade Color"=w63, "PHN"=w61, "Module Info.Customer Number"=w60, "Part Type"=w59) -> (w62:T39)
      }
      frame "Print 60 MBC" {
        n37 = Unbundle By Name(w110) -> ("Module Info.Inalfa Part Number"=w114:string, "Module Info.Serial Number"=w115:string, "Module Info.Sunshade Color"=w117:string, "PHN"=w113:string, "Module Info.Customer Number"=w116:string, "paths.Base Path"=w105:path, "Part Type"=w104:string)
        n38 = call "get path to barcode formats.vi"("product"=w104, "paths.Base Path"=w105) -> ("path"=w106:path)  [unwired: 9 in]
        n39 = call <vilib>:"Check if File or Folder Exists.vi"("error in (no error)"=w103, "path"=w106) -> ("error out"=w107:errorcluster, "file or folder exists?"=w109:bool, "dup path"=w108:path)  [unwired: 7 in]
        n40 = case shown="真" w109 {
          tunnel: w108 -> [_ w124]
          tunnel: w107 -> [w120 w123]
          tunnel: [w120 w122] -> w102
          tunnel: [w119 w121] -> w101
          frame False {
            w119 = T41[] []  # Frame Barcode Formats
          }
          frame True {
            n41 = call "read barcode formats.vi"("error in"=w123, "configuration file path"=w124) -> ("error out"=w122:errorcluster, "Frame Barcode Formats"=w121:T41[])  [unwired: 8 in]
          }
        }
        n42 = call "Barcode Print.vi"("part type"=w104, "Manual?"=TRUE, "error in"=w102, "Part History Number"=w113, "Customer Number"=w116, "Color"=w117, "Serial Number"=w115, "Inalfa Part Number"=w114, "Frame Barcode Formats"=w101) -> ("error out"=w111:errorcluster)  [unwired: 2 in]
      }
      frame "Print Audit MBC" {
        n43 = Unbundle By Name(w141) -> ("paths.Base Path"=w136:path, "Module Info.Inalfa Part Number"=w133:string, "Module Info.Serial Number"=w132:string, "Module Info.Sunshade Color"=w131:string, "Part Type"=w126:string, "PHN"=w130:string, "Module Info.Customer Number"=w129:string)
        n44 = call "get path to audit barcode formats.vi"("product"=w126, "paths.Base Path"=w136) -> ("path"=w137:path)  [unwired: 9 in]
        n45 = call <vilib>:"Check if File or Folder Exists.vi"("error in (no error)"=w135, "path"=w137) -> ("error out"=w138:errorcluster, "file or folder exists?"=w140:bool, "dup path"=w139:path)  [unwired: 7 in]
        n46 = case shown="真" w140 {
          tunnel: w139 -> [_ w148]
          tunnel: w138 -> [w144 w147]
          tunnel: [w144 w146] -> w128
          tunnel: [w143 w145] -> w134
          frame False {
            w143 = T41[] []  # Frame Barcode Formats
          }
          frame True {
            n47 = call "read barcode formats.vi"("error in"=w147, "configuration file path"=w148) -> ("error out"=w146:errorcluster, "Frame Barcode Formats"=w145:T41[])  [unwired: 8 in]
          }
        }
        n48 = call "Barcode Print.vi"("part type"=w126, "Manual?"=TRUE, "error in"=w128, "Part History Number"=w130, "Customer Number"=w129, "Color"=w131, "Serial Number"=w132, "Inalfa Part Number"=w133, "Frame Barcode Formats"=w134) -> ("error out"=w127:errorcluster)  [unwired: 2 in]
      }
      frame "Check Input" {
        n49 = Unbundle By Name(w166) -> ("St 60 MBC Print"=w168:bool, "St 100 MBC Print"=w167:bool, "st60 PLC read boolean Tags.manual barcode print"=w154:T36, "st100 PLC read boolean Tags.manual barcode print"=w150:T36, "Exit Program"=w158:refnum<vi>)
        n50 = property class="Bool (严格)"(reference=w158, error in=w157) -> (error out=w156:errorcluster, "Value"=w155:bool)  [unwired: 1 out]
        n51 = Unbundle By Name(w154) -> ("Tag Name"=w153:string)
        n52 = Unbundle By Name(w150) -> ("Tag Name"=w151:string)
        n53 = Empty String/Path?(string/path=w153) -> (empty?=w152:bool)
        n54 = case shown="假" w152 {
          tunnel: [w177 w179] -> w162
          tunnel: w154 -> [w176 _]
          tunnel: [w175 FALSE ("value")] -> w161
          tunnel: w156 -> [w174 w179]
          frame False {
            n55 = call "plc read bool.vi"("error in"=w174, "addr,tag"=w176) -> ("error out"=w177:errorcluster, "value"=w175:bool)  [unwired: 8 in]
          }
          frame True {
          }
        }
        n56 = Compound Arithmetic op=AND(invert w168, w161) -> (w163:bool)
        n57 = Empty String/Path?(string/path=w151) -> (empty?=w149:bool)
        n58 = case shown="假" w149 {
          tunnel: w162 -> [w183 w185]
          tunnel: w150 -> [w182 _]
          tunnel: [w181 w185] -> w160
          tunnel: [w180 FALSE ("value")] -> w159
          frame False {
            n59 = call "plc read bool.vi"("error in"=w183, "addr,tag"=w182) -> ("error out"=w181:errorcluster, "value"=w180:bool)  [unwired: 8 in]
          }
          frame True {
          }
        }
        n60 = Compound Arithmetic op=AND(invert w167, w159) -> (w164:bool)
        n61 = Build Array(w163, w164, w155) -> (w173:bool[])
        n62 = Search 1D Array(1D array=w173, element=TRUE) -> (index of element=w171:i32)  [unwired: 1 in]
        n63 = Increment(x=w171) -> (x+1=w170:i32)
        n64 = case shown="1" w170 {
          tunnel: [string[] ["Check Input"] ("event queue out") string[] ["Get 60 MBC Info", "Print 60 MBC", "Check Input"] ("event queue out") string[] ["Get Audit MBC Info", "Print Audit MBC", "Check Input"] ("event queue out") string[] ["Exit", "Check Input"] ("event queue out")] -> w169
          frame 0, Default {
          }
          frame 1 {
          }
          frame 2 {
          }
          frame 3 {
          }
        }
        n65 = Bundle By Name(cluster=w166, "St 60 MBC Print"=w161, "St 100 MBC Print"=w159) -> (w165:T39)
      }
    }
  }
  "error out" <- w6
